vi "Create All Data Notifiers.vi"() -> (3 "Initialized Data Notifiers":T1)   [LabVIEW 2013, in "Data Notifiers.lvlib"]
uses:
  Data Notifiers/Data Notifiers.lvlib
  Data Notifiers/All Data Notifiers.ctl
  Acquisition/APD Notifier Cluster.ctl
  Piezo/Piezo display.ctl
  XY/XY Display.ctl
  Capacitive/Capacitive Signal Cluster.ctl
  XY/XY.lvlib
  Desktop/Simon Labview/Piezo.lvlib
  Acquisition/Acquisition.lvlib
  Capacitive/Capacitive.lvlib
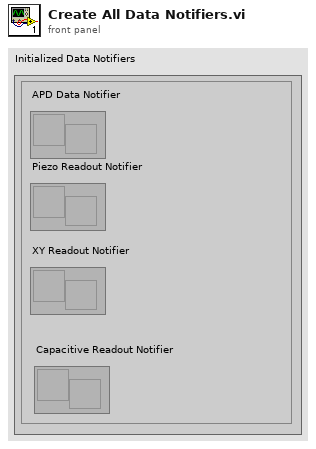
[diagram p1: front panel]
types:
  T1 = typedef "Data Notifiers.lvlib/All Data Notifiers.ctl" = cluster{"APD Data Notifier":refnum<notifier>, "Piezo Readout Notifier":refnum<notifier>, "XY Readout Notifier":refnum<notifier>, "Capacitive Readout Notifier":refnum<notifier>}
  T2 = typedef "Capacitive.lvlib/Capacitive Signal Cluster.ctl" = cluster{"Readout":sgl, "Time":i32}
  T3 = typedef "Acquisition.lvlib/APD Notifier Cluster.ctl" = cluster{"data":dbl[], "t0":i32}
  T4 = typedef "Piezo.lvlib/Piezo display.ctl" = cluster{"PiezoPosition":sgl, "Counter Time":i32}
  T5 = typedef "XY.lvlib/XY Display.ctl" = cluster{"X Position":sgl, "Y Position":sgl}
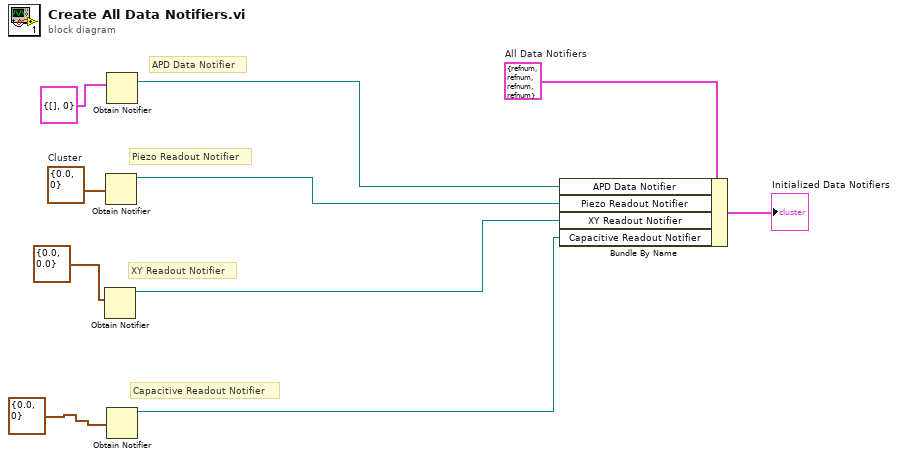
[diagram p0: block diagram]
diagram:
  w6 = T1 {"APD Data Notifier"=refnum, "Piezo Readout Notifier"=refnum, "XY Readout Notifier"=refnum, "Capacitive Readout Notifier"=refnum}  # All Data Notifiers
  w10 = T4 {"PiezoPosition"=0.0, "Counter Time"=0}  # Cluster
  # "Capacitive Readout Notifier"
  # "XY Readout Notifier"
  # "Piezo Readout Notifier"
  # "APD Data Notifier"
  n1 = Obtain Notifier(notification data type=T5 {"X Position"=0.0, "Y Position"=0.0} ("Cluster")) -> (notifier out=w4:refnum<notifier>)  [unwired: 3 in, 2 out]
  n2 = Obtain Notifier(notification data type=w10) -> (notifier out=w5:refnum<notifier>)  [unwired: 3 in, 2 out]
  n3 = Obtain Notifier(notification data type=T3 {"data"=[], "t0"=0}) -> (notifier out=w7:refnum<notifier>)  [unwired: 3 in, 2 out]
  n4 = Obtain Notifier(notification data type=T2 {"Readout"=0.0, "Time"=0} ("Capacitive Signal Cluster")) -> (notifier out=w3:refnum<notifier>)  [unwired: 3 in, 2 out]
  n5 = Bundle By Name(cluster=w6, "APD Data Notifier"=w7, "Piezo Readout Notifier"=w5, "XY Readout Notifier"=w4, "Capacitive Readout Notifier"=w3) -> (→"Initialized Data Notifiers":T1)
